vi "FWCS.vi"() -> ()   [LabVIEW 2018]
uses:
  Roda_Filtros/Roda_Filtros.lvclass
  SIM_Roda_Filtros/SIM_Roda_Filtros.lvclass
  C:/Users/observer/Desktop/FWCS/FWCS/Roda_Filtros/Roda_Filtros.lvclass
  Roda_Filtros/Roda_Filtros.lvclass/Roda_Filtros.ctl
panel:
  in  "Real/Simulated":bool
  in  "Remote IP":string="200.131.64.49"
  out "Current Filter":u16(ring)=1 items=["U"=1, "B"=2, "V"=3, "R"=4, "I"=5, "Clear"=6]
  in  "Serial Port":string="COM6"
  in  "Select Filter":u16(ring)=1 items=["U"=1, "B"=2, "V"=3, "R"=4, "I"=5, "Clear"=6]
  out "Error message":string
  in  "stop":bool
  out "communication status":bool
  # "Filter Wheel Control System (FWCS)"
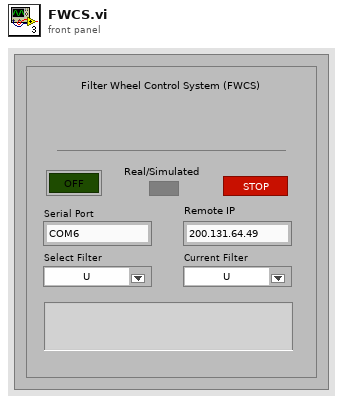
[diagram p1: front panel]
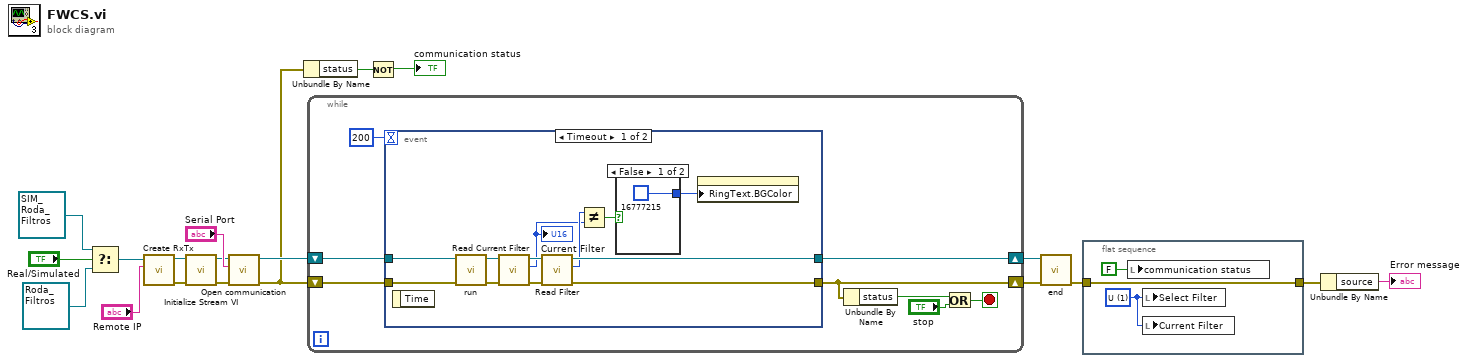
[diagram p0: block diagram]
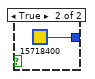
[diagram p2: hidden frame]
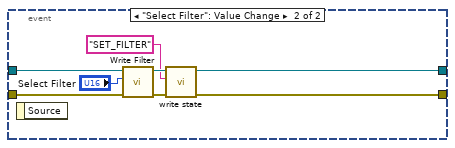
[diagram p3: hidden frame]
diagram:
  n1 = Select(t=refnum<class "SIM_Roda_Filtros.lvclass"> refnum ("SIM_Roda_Filtros.lvclass"), s="Real/Simulated", f=refnum<class "Roda_Filtros.lvclass"> refnum ("Roda_Filtros in")) -> (s? t:f=w1:refnum<class "Roda_Filtros.lvclass">)
  n2 = call "Create RxTx.vi"("Remote IP"="Remote IP", "Roda_Filtros in"=w1) -> ("error out"=w9:errorcluster, "Roda_Filtros out"=w10:refnum<class "Roda_Filtros.lvclass">)  [unwired: 8 in]
  n3 = call "Initialize Stream VI.vi"("error in (no error)"=w9, "Roda_Filtros in"=w10) -> ("error out"=w11:errorcluster, "Roda_Filtros out"=w12:refnum<class "Roda_Filtros.lvclass">)  [unwired: 8 in]
  n4 = call-dynamic "Open communication.vi"("error in (no error)"=w11, "port"="Serial Port", "Roda_Filtros in"=w12) -> ("error out"=w8:errorcluster, "Roda_Filtros out"=w18:refnum<class "Roda_Filtros.lvclass">)  [unwired: 6 in, 1 out]
  n5 = Unbundle By Name(w8) -> ("status"=w7:bool)
  n6 = while {
    shift-right: [w21] -> w13
    shift-left: w18 -> [w26]
    shift-right: [w25] -> w14
    shift-left: w8 -> [w27]
    stop <- w22 stop-if-true
    n7 = event shown="[0] Timeout" {
      selector: _ -> [_ _]
      dyn-events: _ -> [_ _]
      timeout: 200 -> [_ _]
      tunnel: w27 -> [w38 w48]
      tunnel: w26 -> [w39 w49]
      tunnel: [w33 w44] -> w25
      tunnel: [w32 w45] -> w21
      event Timeout {
        n8 = event-data() -> ()  [unwired: 1 in, 1 out]
        n9 = call "run.vi"("error in (no error)"=w38, "Roda_Filtros in"=w39) -> ("error out"=w37:errorcluster, "Roda_Filtros out"=w36:refnum<class "Roda_Filtros.lvclass">)  [unwired: 8 in]
        n10 = call "Read Current Filter.vi"("error in (no error)"=w37, "Roda_Filtros in"=w36) -> ("error out"=w34:errorcluster, "Current Filter"=w29:u16, "Roda_Filtros out"=w35:refnum<class "Roda_Filtros.lvclass">)  [unwired: 7 in]
        "Current Filter" <- w29
        n11 = call "Read Filter.vi"("error in (no error)"=w34, "Roda_Filtros in"=w35) -> ("error out"=w33:errorcluster, "Filter"=w30:u16, "Roda_Filtros out"=w32:refnum<class "Roda_Filtros.lvclass">)  [unwired: 7 in]
        n12 = Not Equal?(x=w30, y=w29) -> (x != y?=w31:bool)
        n13 = case shown="False" w31 {
          tunnel: [u32 16777215 u32 15718400] -> w28
          frame False {
          }
          frame True {
          }
        }
        n14 = property on="Current Filter" class="Ring (strict)"("RingText.BGColor"=w28) -> ()  [unwired: 2 in, 2 out]
      }
      event "Select Filter": Value Change {
        n15 = event-data() -> ()  [unwired: 1 in, 1 out]
        n16 = call "Write Filter.vi"("error in (no error)"=w48, "Filter"="Select Filter", "Roda_Filtros in"=w49) -> ("error out"=w43:errorcluster, "Roda_Filtros out"=w46:refnum<class "Roda_Filtros.lvclass">)  [unwired: 7 in]
        n17 = call "write state.vi"("error in (no error)"=w43, "State"="SET_FILTER", "Roda_Filtros in"=w46) -> ("error out"=w44:errorcluster, "Roda_Filtros out"=w45:refnum<class "Roda_Filtros.lvclass">)  [unwired: 7 in]
      }
    }
    n18 = Unbundle By Name(w25) -> ("status"=w24:bool)
    n19 = Or(x=w24, y="stop") -> (x .or. y?=w22:bool)
  }
  n20 = Not(x=w7) -> (.not. x?=→"communication status":bool)
  n21 = call "end.vi"("error in (no error)"=w14, "Roda_Filtros in"=w13) -> ("error out"=w15:errorcluster)  [unwired: 8 in, 1 out]
  n22 = flat-sequence {
    tunnel: w15 -> [w52]
    tunnel: [w52] -> w17
    frame #0 {
      w50 = u16 1 items=["U"=1, "B"=2, "V"=3, "R"=4, "I"=5, "Clear"=6] ("Select Filter")
      n23 = local write "communication status"(FALSE ("communication status")) -> ()
      n24 = local write "Select Filter"(w50) -> ()
      n25 = local write "Current Filter"(w50) -> ()
    }
  }
  n26 = Unbundle By Name(w17) -> ("source"=→"Error message":string)
